vi "Tom_remove.vi"(8 "Flip Hammer":bool, 9 "XScale.Minimum":dbl, 10 "XScale.Maximum":dbl, 11 "Data in":waveform(dbl)[](array[waveform])) -> (2 "Removed":waveform(dbl)[](array[waveform]), 3 "Cleaned":waveform(dbl)[](array[waveform]))   [LabVIEW 2024]
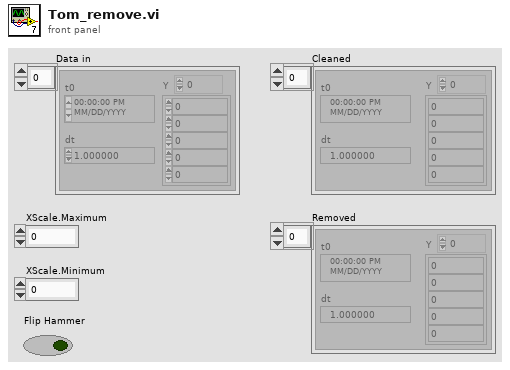
[diagram p1: front panel]
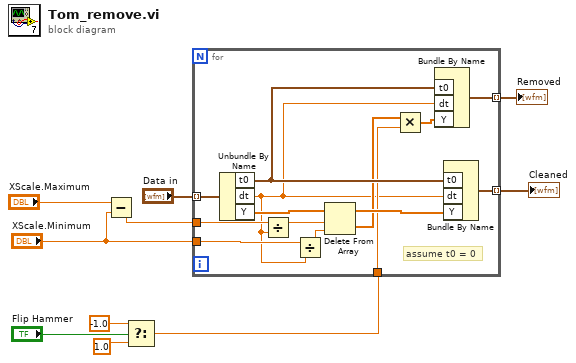
[diagram p0: block diagram]
diagram:
  n1 = Subtract(x="XScale.Maximum", y="XScale.Minimum") -> (x-y=w1:dbl)
  n2 = Select(t=-1.0, s="Flip Hammer", f=1.0 ("t")) -> (s? t:f=w3:dbl)
  n3 = for {
    tunnel: "Data in" -> [w24] mode=indexing
    tunnel: "XScale.Minimum" -> [w14]
    tunnel: w1 -> [w21]
    tunnel: [w20] -> w9 mode=indexing
    tunnel: [w19] -> w10 mode=indexing
    tunnel: w3 -> [w17]
    # "assume t0 = 0"
    n4 = Unbundle By Name(w24) -> ("t0"=w18:timestamp, "dt"=w13:dbl, "Y"=w23:dbl[])
    n5 = Divide(x=w21, y=w13) -> (x/y=w12:dbl)
    n6 = Divide(x=w14, y=w13) -> (x/y=w11:dbl)
    n7 = Delete From Array(array=w23, length=w12, index=w11) -> (deleted portion=w16:dbl[], array with subset deleted=w22:dbl[])
    n8 = Multiply(x=w16, y=w17) -> (x*y=w15:dbl[])
    n9 = Bundle By Name("t0"=w18, "dt"=w13, "Y"=w15) -> (w19:waveform(dbl))  [unwired: 1 in]
    n10 = Bundle By Name("t0"=w18, "dt"=w13, "Y"=w22) -> (w20:waveform(dbl))  [unwired: 1 in]
  }
  "Removed" <- w10
  "Cleaned" <- w9
